vi "Pre-Loader.vi"(8 "error in (no error)":errorcluster) -> (0 "error out":errorcluster, 3 "Cancel?":bool)   [LabVIEW 2021, in "User Interface.lvlib"]
uses:
  User Interface.lvlib
  Pre-Loader Command.ctl
  CVT/Input Command.ctl
  Database/Database.lvlib
  DAQ Hardware/DAQ Hardware.lvlib
  DAQ IO/DAQ IO.lvlib
  ARINC/ARINC.lvlib
  S-Matrix/S-Matrix.lvlib
  DC PWS/DC PWS.lvlib
  DMM/DMM.lvlib
  Func Generator/Func Generator.lvlib
  Oscilloscope/Oscilloscope.lvlib
  Environment Chamber/Environment Chamber.lvlib
  CVT/CVT.lvlib
  CAN/CAN.lvlib
panel:
  out "Exit?":bool
  out "Title?":string="Pre-Loader"
  out "Msg":string
  out "Slider":i32(slide) scale=0.0..10.0
  in  "Stop":bool
  out "Time":string="Sat  8/3/2019  8:10:44 PM"
  # "21/511, Hosur Rd, Electronic City, Phase 1,Bengaluru, Karnataka 560100"
  # "21/511, Hosur Rd, Lavakusha Nagar, 1st Phase, Electronic City, Bengaluru, Karnataka 560100"
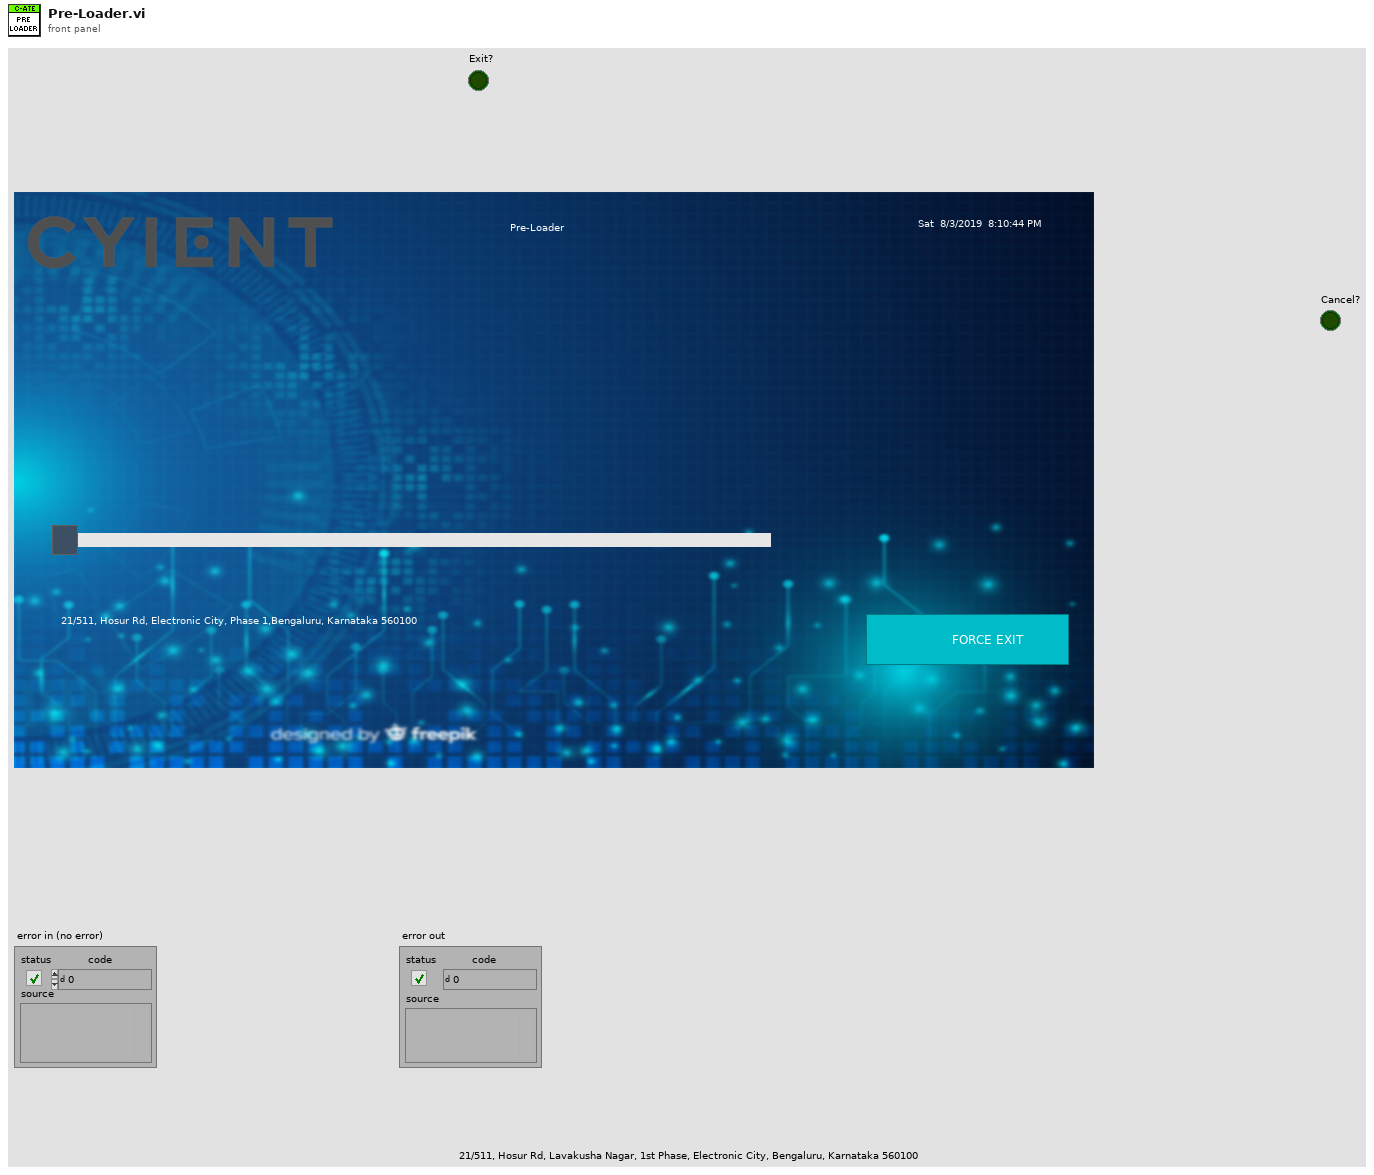
[diagram p1: front panel]
types:
  T1 = typedef "User Interface.lvlib/Pre-Loader Command.ctl" = enum16{"Init", "Check Database", "Check NI DAQ", "Check NI DIO", "Check CAN", "Check ARINC", "Check Matrix", "Check DC Power Supply", "Check DMM", "Check Function Gen", "Check Oscilloscope", "Check ESPEC", "Check CVT", "Exit"}
  T2 = typedef "CVT.lvlib/Input Command.ctl" = enum16{"DC PWS", "DMM", "FGEN", "Oscill", "NI DAQ", "NI DIO", "NI CAN", "ESPEC", "ARINC", "MATRIX", "CVT"}
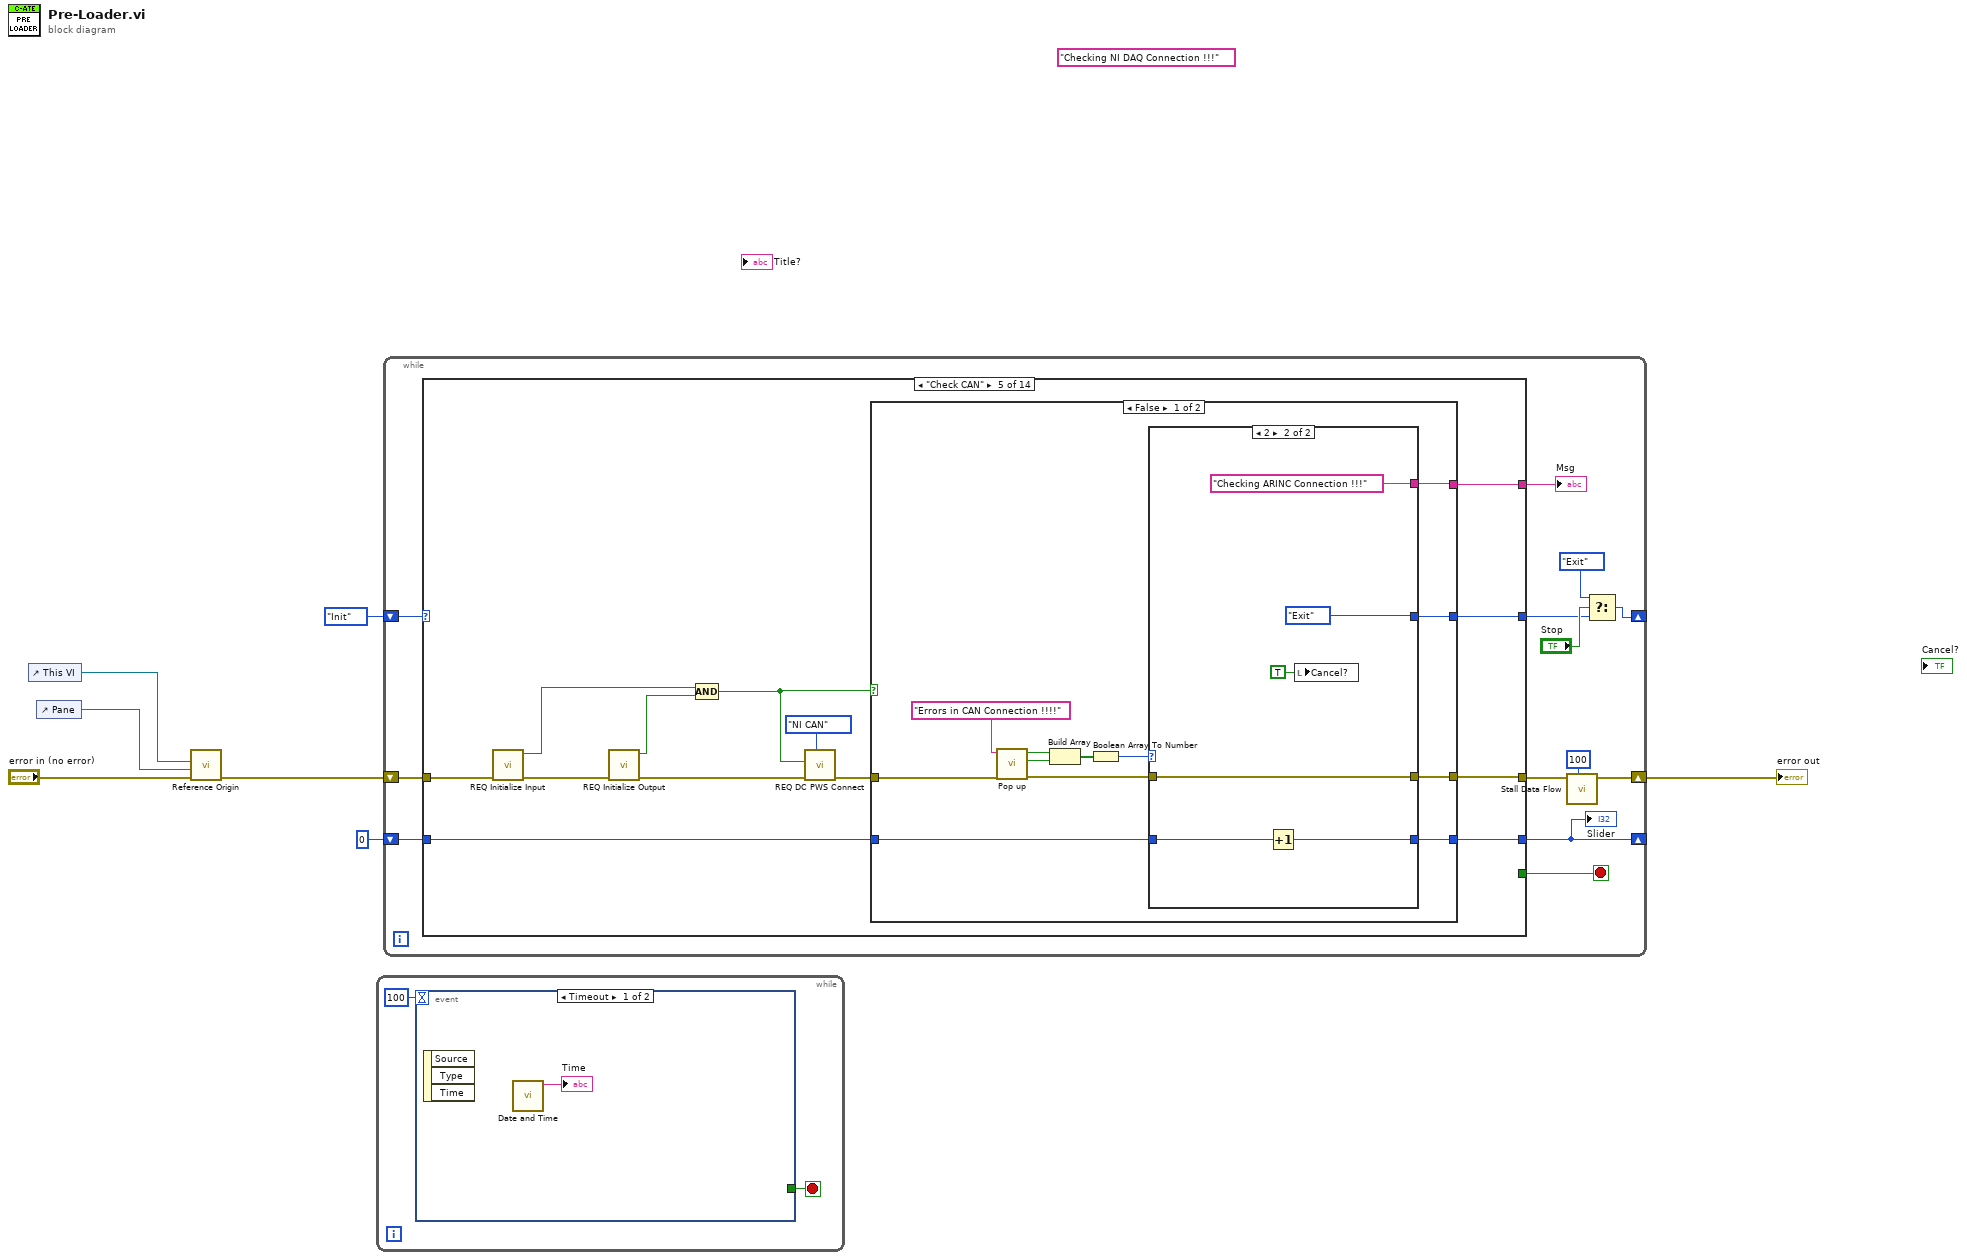
[diagram p0: block diagram]
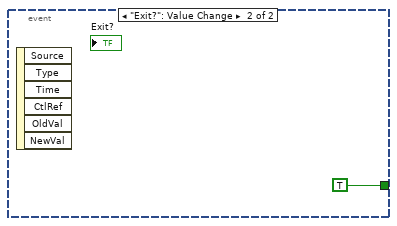
[diagram p2: hidden frame]
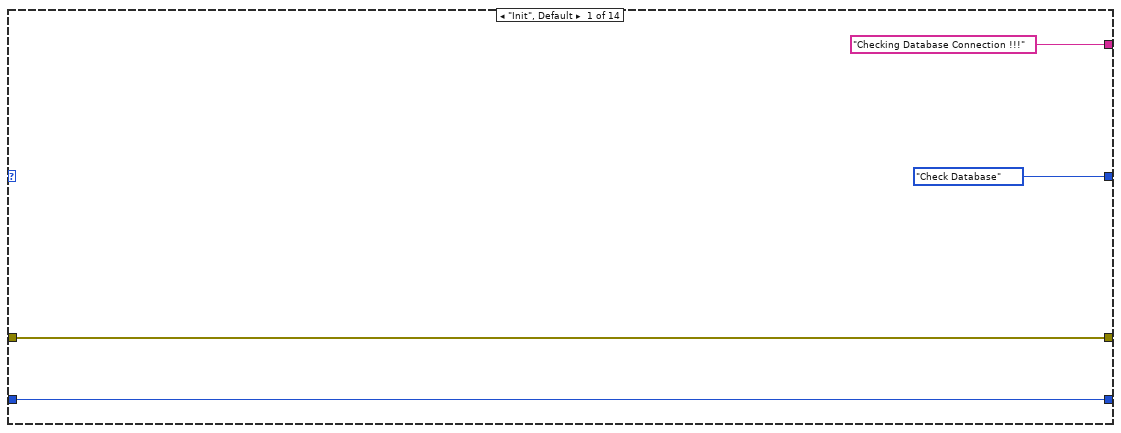
[diagram p3: hidden frame]
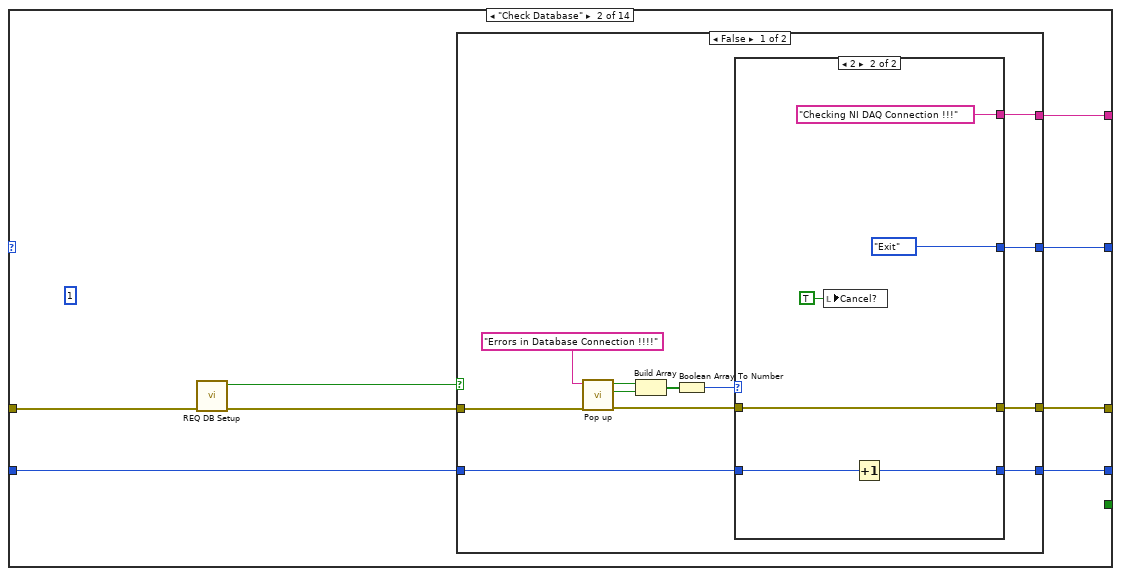
[diagram p4: hidden frame]
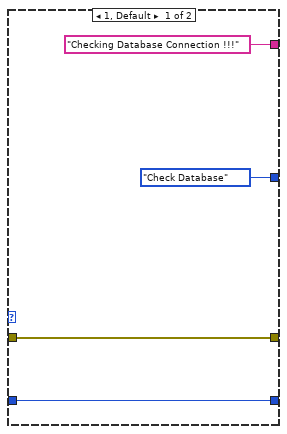
[diagram p5: hidden frame]
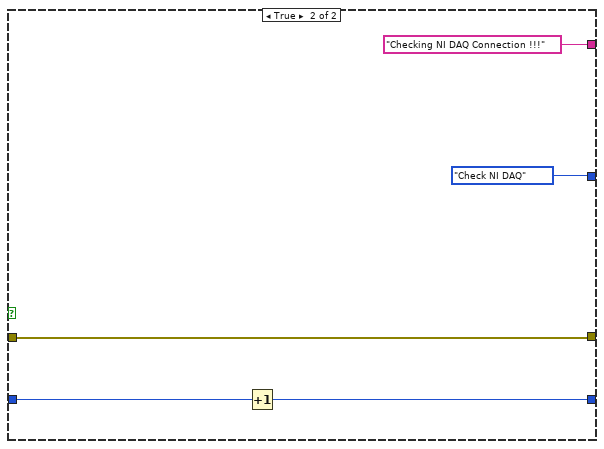
[diagram p6: hidden frame]
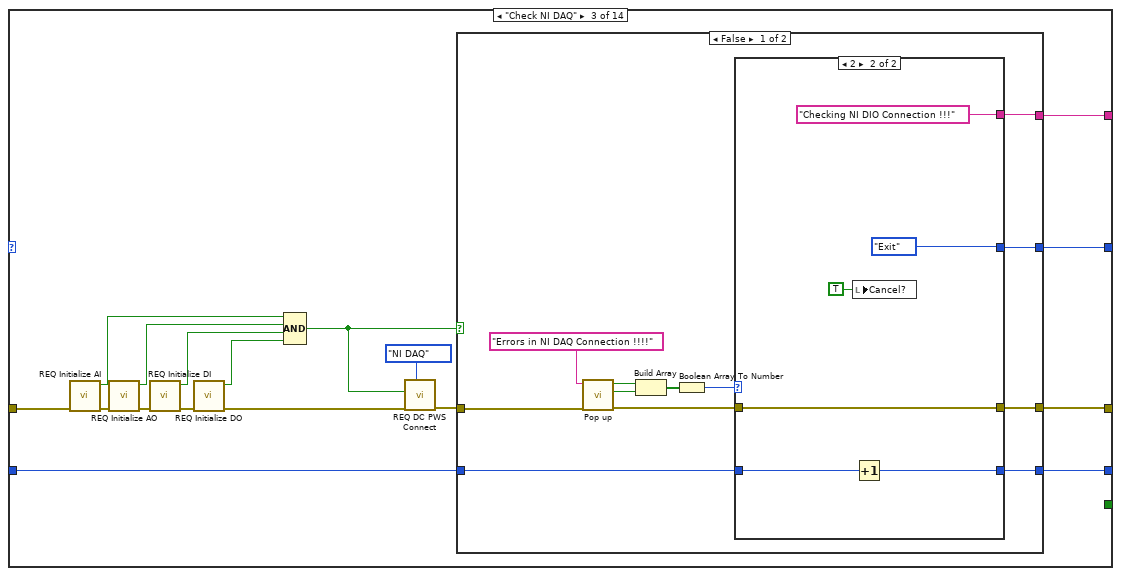
[diagram p7: hidden frame]
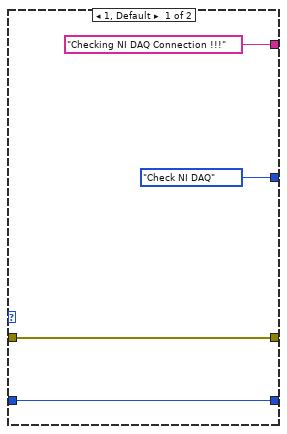
[diagram p8: hidden frame]
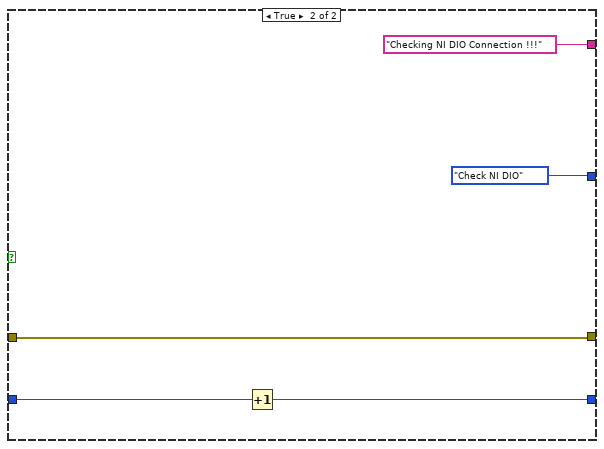
[diagram p9: hidden frame]
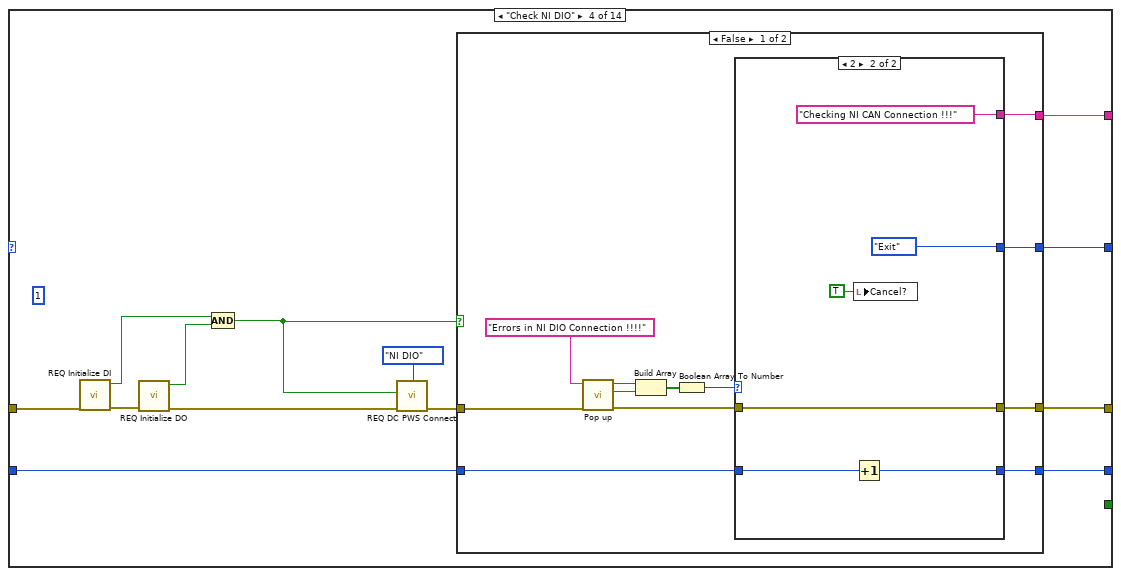
[diagram p10: hidden frame]
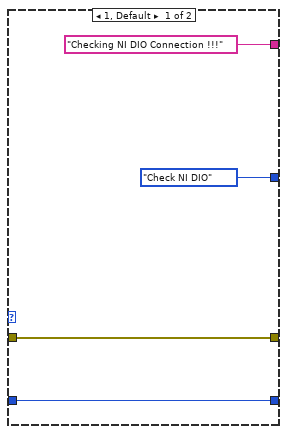
[diagram p11: hidden frame]
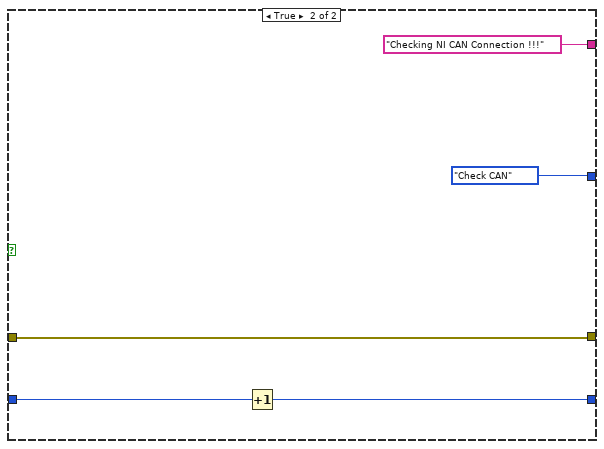
[diagram p12: hidden frame]
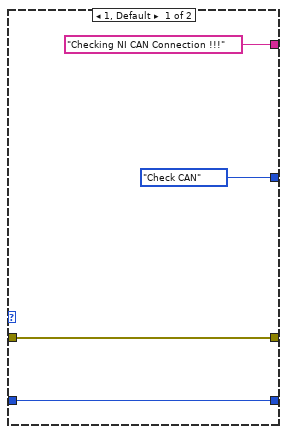
[diagram p13: hidden frame]
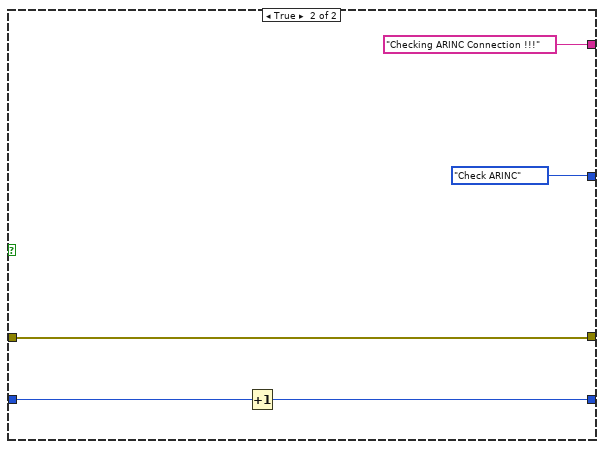
[diagram p14: hidden frame]
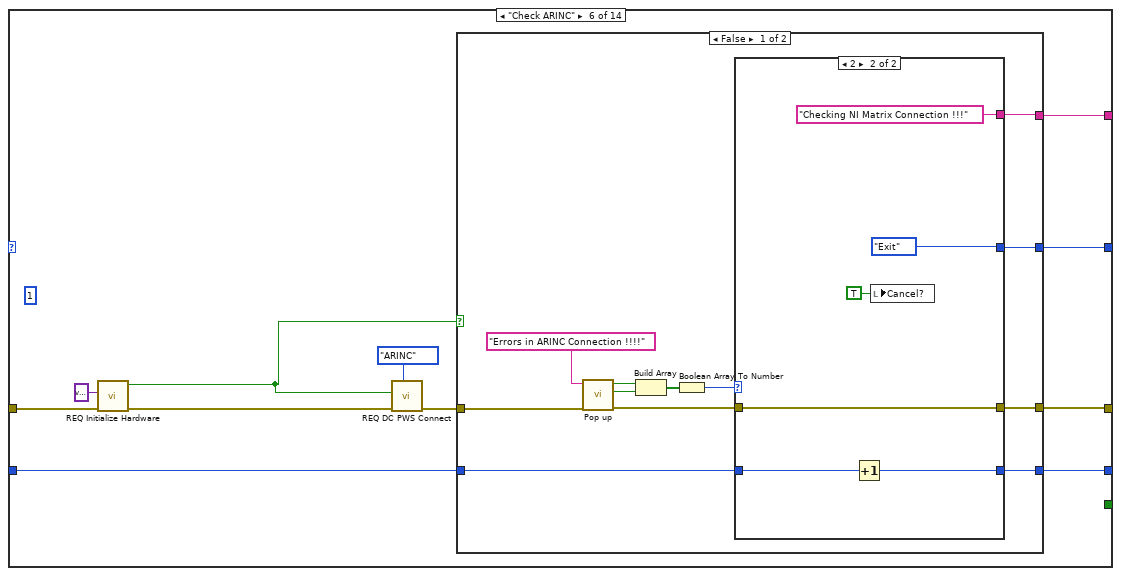
[diagram p15: hidden frame]
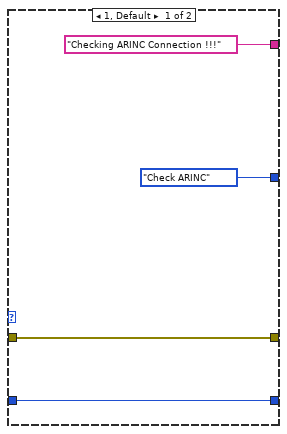
[diagram p16: hidden frame]
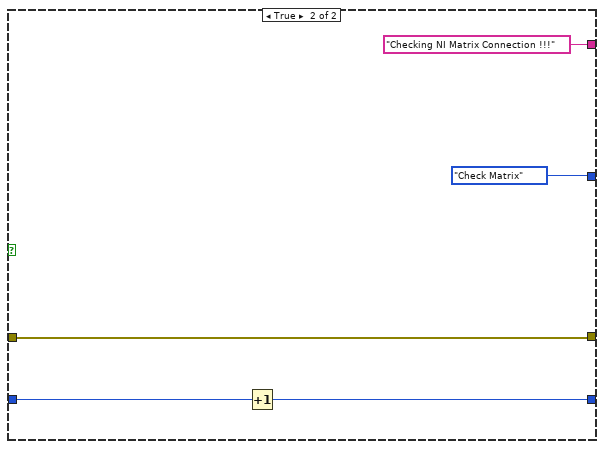
[diagram p17: hidden frame]
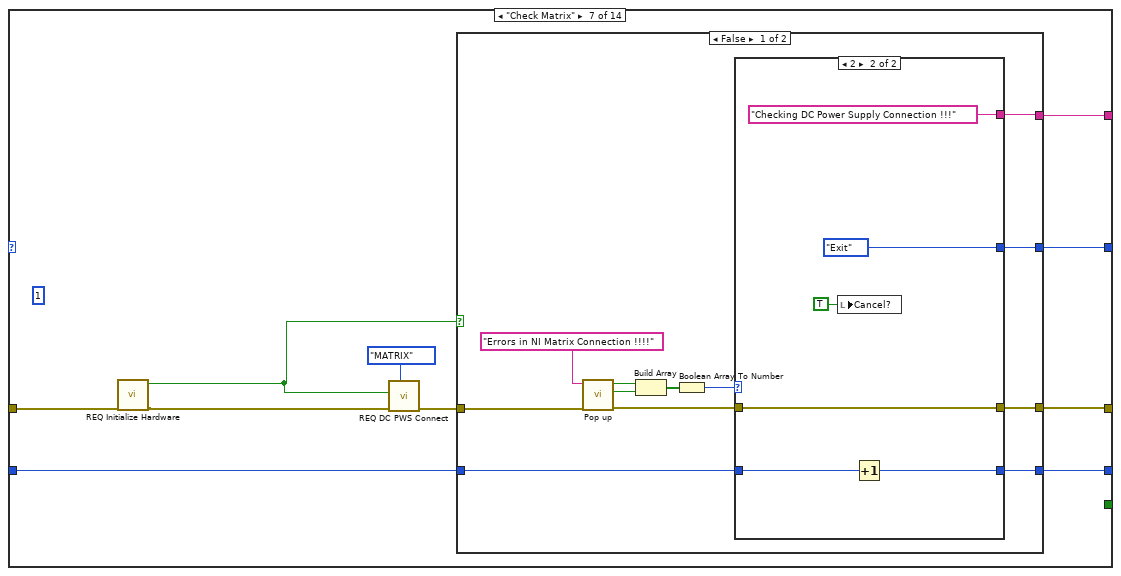
[diagram p18: hidden frame]
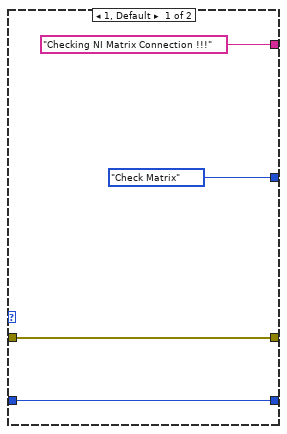
[diagram p19: hidden frame]
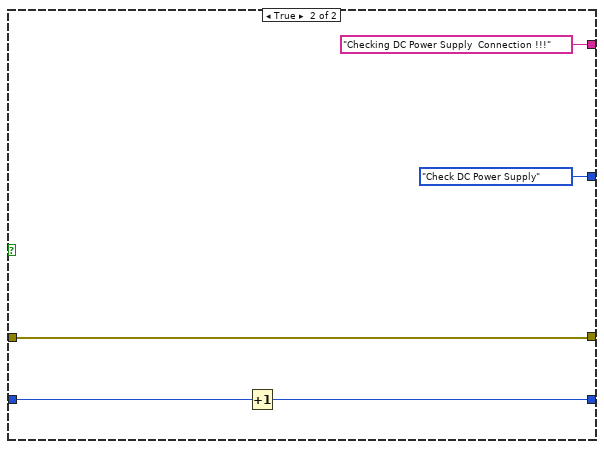
[diagram p20: hidden frame]
diagram:
  (unwired) "Checking NI DAQ Connection !!!"
  n1 = control-ref of="This VI"() -> (w6:refnum<vi>)
  n2 = control-ref of="Pane"() -> (w5:refnum<vi>)
  n3 = call "Reference Origin.vi"("error in (no error)"="error in (no error)", "Pane"=w5, "This VI"=w6) -> ("error out"=w4:errorcluster)  [unwired: 8 in]
  n4 = while {
    stop <- w8 stop-if-true
    n5 = event shown="[0] Timeout" {
      selector: _ -> [_ _]
      dyn-events: _ -> [_ _]
      timeout: 100 -> [_ _]
      tunnel: [_ TRUE] -> w8
      event Timeout {
        n6 = event-data() -> ()  [unwired: 1 in, 3 out]
        n7 = call "Date and Time.vi"() -> ("Current Time"=→"Time":string)  [unwired: 11 in]
      }
      event "Exit?": Value Change {
        n8 = event-data() -> ()  [unwired: 1 in, 6 out]
      }
    }
  }
  n9 = while {
    shift-right: [w20] -> _
    shift-left: Pre-Loader_Command."Init" -> [w24]
    shift-right: [w12] -> _
    shift-left: 0 -> [w13]
    shift-right: [w15] -> w3
    shift-left: w4 -> [w16]
    stop <- w18 stop-if-true
    n10 = case shown="\"Check CAN\"" w24 {
      tunnel: ["Checking Database Connection !!!" w29 w75 w115 w156 w193 w230 w267 w304 w341 w379 w417 w455 _] -> w23
      tunnel: [Pre-Loader_Command."Check Database" w30 w76 w116 w157 w194 w231 w268 w305 w342 w380 w418 w456 Pre-Loader_Command."Exit"] -> w21
      tunnel: [_ _ _ _ _ _ _ _ _ _ _ _ _ TRUE] -> w18
      tunnel: [w26 w33 w79 w119 w160 w197 w234 w271 w308 w345 w383 w421 w459 w487] -> w17
      tunnel: w16 -> [w26 w36 w80 w120 w153 w198 w235 w272 w309 w346 w384 w422 w452 w489]
      tunnel: w13 -> [w25 w32 w78 w118 w159 w196 w233 w270 w307 w344 w382 w420 w458 w491]
      tunnel: [w25 w31 w77 w117 w158 w195 w232 w269 w306 w343 w381 w419 w457 w491] -> w12
      frame "Init", Default {
      }
      frame "Check Database" {
        (unwired) 1
        n11 = call "REQ DB Setup.vi"("error in"=w36) -> ("error out"=w35:errorcluster, "Connect?"=w34:bool)  [unwired: 8 in, 1 out]
        n12 = case shown="False" w34 {
          tunnel: w35 -> [w48 w61]
          tunnel: [w39 w61] -> w33
          tunnel: w32 -> [w38 w63]
          tunnel: [w37 w62] -> w31
          tunnel: [w40 Pre-Loader_Command."Check NI DAQ"] -> w30
          tunnel: [w41 "Checking NI DAQ Connection !!!"] -> w29
          frame False {
            n13 = call "Pop up.vi"("error in (no error)"=w48, "Message In"="Errors in Database Connection !!!!") -> ("error out"=w42:errorcluster, "Next?"=w45:bool, "Retry?"=w46:bool)  [unwired: 7 in]
            n14 = Build Array(w46, w45) -> (w44:bool[])
            n15 = Boolean Array To Number(Boolean array=w44) -> (number=w43:u32)
            n16 = case shown="2" w43 {
              tunnel: w42 -> [w50 w56]
              tunnel: ["Checking Database Connection !!!" "Checking NI DAQ Connection !!!"] -> w41
              tunnel: [Pre-Loader_Command."Check Database" Pre-Loader_Command."Exit"] -> w40
              tunnel: [w50 w56] -> w39
              tunnel: w38 -> [w49 w55]
              tunnel: [w49 w54] -> w37
              frame 1, Default {
              }
              frame 2 {
                n17 = local write "Cancel?"(TRUE ("Cancel?")) -> ()
                n18 = Increment(x=w55) -> (x+1=w54:i32)
              }
            }
          }
          frame True {
            n19 = Increment(x=w63) -> (x+1=w62:i32)
          }
        }
      }
      frame "Check NI DAQ" {
        n20 = call "REQ Initialize AI.vi"("error in"=w80) -> ("error out"=w71:errorcluster, "Connect?"=w68:bool)  [unwired: 8 in, 1 out]
        n21 = call "REQ Initialize AO.vi"("error in"=w71) -> ("error out"=w70:errorcluster, "Connect?"=w67:bool)  [unwired: 8 in, 1 out]
        n22 = call "REQ Initialize DI.vi"("error in"=w70) -> ("error out"=w69:errorcluster, "Connect?"=w66:bool)  [unwired: 8 in, 1 out]
        n23 = call "REQ Initialize DO.vi"("error in"=w69) -> ("error out"=w73:errorcluster, "Connect?"=w65:bool)  [unwired: 8 in, 1 out]
        n24 = Compound Arithmetic op=AND(w68, w67, w66, w65) -> (w64:bool)
        n25 = call "REQ DC PWS Connect.vi"("Command"=Input_Command."NI DAQ", "error in"=w73, "Connect ?"=w64) -> ("error out"=w72:errorcluster)  [unwired: 8 in]
        n26 = case shown="False" w64 {
          tunnel: w72 -> [w92 w105]
          tunnel: [w83 w105] -> w79
          tunnel: w78 -> [w82 w107]
          tunnel: [w81 w106] -> w77
          tunnel: [w84 Pre-Loader_Command."Check NI DIO"] -> w76
          tunnel: [w85 "Checking NI DIO Connection !!!"] -> w75
          frame False {
            n27 = call "Pop up.vi"("error in (no error)"=w92, "Message In"="Errors in NI DAQ Connection !!!!") -> ("error out"=w86:errorcluster, "Next?"=w89:bool, "Retry?"=w90:bool)  [unwired: 7 in]
            n28 = Build Array(w90, w89) -> (w88:bool[])
            n29 = Boolean Array To Number(Boolean array=w88) -> (number=w87:u32)
            n30 = case shown="2" w87 {
              tunnel: w86 -> [w94 w100]
              tunnel: ["Checking NI DAQ Connection !!!" "Checking NI DIO Connection !!!"] -> w85
              tunnel: [Pre-Loader_Command."Check NI DAQ" Pre-Loader_Command."Exit"] -> w84
              tunnel: [w94 w100] -> w83
              tunnel: w82 -> [w93 w99]
              tunnel: [w93 w98] -> w81
              frame 1, Default {
              }
              frame 2 {
                n31 = local write "Cancel?"(TRUE ("Cancel?")) -> ()
                n32 = Increment(x=w99) -> (x+1=w98:i32)
              }
            }
          }
          frame True {
            n33 = Increment(x=w107) -> (x+1=w106:i32)
          }
        }
      }
      frame "Check NI DIO" {
        (unwired) 1
        n34 = call "REQ Initialize DI.vi"("error in"=w120) -> ("error out"=w110:errorcluster, "Connect?"=w108:bool)  [unwired: 8 in, 1 out]
        n35 = call "REQ Initialize DO.vi"("error in"=w110) -> ("error out"=w113:errorcluster, "Connect?"=w109:bool)  [unwired: 8 in, 1 out]
        n36 = Compound Arithmetic op=AND(w108, w109) -> (w111:bool)
        n37 = call "REQ DC PWS Connect.vi"("Command"=Input_Command."NI DIO", "error in"=w113, "Connect ?"=w111) -> ("error out"=w112:errorcluster)  [unwired: 8 in]
        n38 = case shown="False" w111 {
          tunnel: w112 -> [w132 w145]
          tunnel: [w123 w145] -> w119
          tunnel: w118 -> [w122 w147]
          tunnel: [w121 w146] -> w117
          tunnel: [w124 Pre-Loader_Command."Check CAN"] -> w116
          tunnel: [w125 "Checking NI CAN Connection !!!"] -> w115
          frame False {
            n39 = call "Pop up.vi"("error in (no error)"=w132, "Message In"="Errors in NI DIO Connection !!!!") -> ("error out"=w126:errorcluster, "Next?"=w129:bool, "Retry?"=w130:bool)  [unwired: 7 in]
            n40 = Build Array(w130, w129) -> (w128:bool[])
            n41 = Boolean Array To Number(Boolean array=w128) -> (number=w127:u32)
            n42 = case shown="2" w127 {
              tunnel: w126 -> [w134 w140]
              tunnel: ["Checking NI DIO Connection !!!" "Checking NI CAN Connection !!!"] -> w125
              tunnel: [Pre-Loader_Command."Check NI DIO" Pre-Loader_Command."Exit"] -> w124
              tunnel: [w134 w140] -> w123
              tunnel: w122 -> [w133 w139]
              tunnel: [w133 w138] -> w121
              frame 1, Default {
              }
              frame 2 {
                n43 = local write "Cancel?"(TRUE ("Cancel?")) -> ()
                n44 = Increment(x=w139) -> (x+1=w138:i32)
              }
            }
          }
          frame True {
            n45 = Increment(x=w147) -> (x+1=w146:i32)
          }
        }
      }
      frame "Check CAN" {
        n46 = call "REQ Initialize Input.vi"("error in"=w153) -> ("error out"=w152:errorcluster, "Connect?"=w150:bool)  [unwired: 8 in, 1 out]
        n47 = call "REQ Initialize Output.vi"("error in"=w152) -> ("error out"=w151:errorcluster, "Connect?"=w149:bool)  [unwired: 8 in, 1 out]
        n48 = Compound Arithmetic op=AND(w150, w149) -> (w148:bool)
        n49 = call "REQ DC PWS Connect.vi"("Command"=Input_Command."NI CAN", "error in"=w151, "Connect ?"=w148) -> ("error out"=w154:errorcluster)  [unwired: 8 in]
        n50 = case shown="False" w148 {
          tunnel: w154 -> [w172 w185]
          tunnel: [w163 w185] -> w160
          tunnel: w159 -> [w162 w187]
          tunnel: [w161 w186] -> w158
          tunnel: [w164 Pre-Loader_Command."Check ARINC"] -> w157
          tunnel: [w165 "Checking ARINC Connection !!!"] -> w156
          frame False {
            n51 = call "Pop up.vi"("error in (no error)"=w172, "Message In"="Errors in CAN Connection !!!!") -> ("error out"=w166:errorcluster, "Next?"=w169:bool, "Retry?"=w170:bool)  [unwired: 7 in]
            n52 = Build Array(w170, w169) -> (w168:bool[])
            n53 = Boolean Array To Number(Boolean array=w168) -> (number=w167:u32)
            n54 = case shown="2" w167 {
              tunnel: w166 -> [w174 w180]
              tunnel: ["Checking NI CAN Connection !!!" "Checking ARINC Connection !!!"] -> w165
              tunnel: [Pre-Loader_Command."Check CAN" Pre-Loader_Command."Exit"] -> w164
              tunnel: [w174 w180] -> w163
              tunnel: w162 -> [w173 w179]
              tunnel: [w173 w178] -> w161
              frame 1, Default {
              }
              frame 2 {
                n55 = Increment(x=w179) -> (x+1=w178:i32)
                n56 = local write "Cancel?"(TRUE ("Cancel?")) -> ()
              }
            }
          }
          frame True {
            n57 = Increment(x=w187) -> (x+1=w186:i32)
          }
        }
      }
      frame "Check ARINC" {
        (unwired) 1
        n58 = call "REQ Initialize Hardware.vi"("error in"=w198, "Connection Ref"=variant) -> ("error out"=w191:errorcluster, "Connect?"=w189:bool)  [unwired: 7 in, 1 out]
        n59 = call "REQ DC PWS Connect.vi"("Command"=Input_Command."ARINC", "error in"=w191, "Connect ?"=w189) -> ("error out"=w190:errorcluster)  [unwired: 8 in]
        n60 = case shown="False" w189 {
          tunnel: w190 -> [w210 w223]
          tunnel: [w201 w223] -> w197
          tunnel: w196 -> [w200 w225]
          tunnel: [w199 w224] -> w195
          tunnel: [w202 Pre-Loader_Command."Check Matrix"] -> w194
          tunnel: [w203 "Checking NI Matrix Connection !!!"] -> w193
          frame False {
            n61 = call "Pop up.vi"("error in (no error)"=w210, "Message In"="Errors in ARINC Connection !!!!") -> ("error out"=w204:errorcluster, "Next?"=w207:bool, "Retry?"=w208:bool)  [unwired: 7 in]
            n62 = Build Array(w208, w207) -> (w206:bool[])
            n63 = Boolean Array To Number(Boolean array=w206) -> (number=w205:u32)
            n64 = case shown="2" w205 {
              tunnel: w204 -> [w212 w218]
              tunnel: ["Checking ARINC Connection !!!" "Checking NI Matrix Connection !!!"] -> w203
              tunnel: [Pre-Loader_Command."Check ARINC" Pre-Loader_Command."Exit"] -> w202
              tunnel: [w212 w218] -> w201
              tunnel: w200 -> [w211 w217]
              tunnel: [w211 w216] -> w199
              frame 1, Default {
              }
              frame 2 {
                n65 = Increment(x=w217) -> (x+1=w216:i32)
                n66 = local write "Cancel?"(TRUE ("Cancel?")) -> ()
              }
            }
          }
          frame True {
            n67 = Increment(x=w225) -> (x+1=w224:i32)
          }
        }
      }
      frame "Check Matrix" {
        (unwired) 1
        n68 = call "REQ Initialize Hardware.vi"("error in"=w235) -> ("error out"=w228:errorcluster, "Connect?"=w226:bool)  [unwired: 8 in, 1 out]
        n69 = call "REQ DC PWS Connect.vi"("Command"=Input_Command."MATRIX", "error in"=w228, "Connect ?"=w226) -> ("error out"=w227:errorcluster)  [unwired: 8 in]
        n70 = case shown="False" w226 {
          tunnel: w227 -> [w247 w260]
          tunnel: [w238 w260] -> w234
          tunnel: w233 -> [w237 w262]
          tunnel: [w236 w261] -> w232
          tunnel: [w239 Pre-Loader_Command."Check DC Power Supply"] -> w231
          tunnel: [w240 "Checking DC Power Supply  Connection !!!"] -> w230
          frame False {
            n71 = call "Pop up.vi"("error in (no error)"=w247, "Message In"="Errors in NI Matrix Connection !!!!") -> ("error out"=w241:errorcluster, "Next?"=w244:bool, "Retry?"=w245:bool)  [unwired: 7 in]
            n72 = Build Array(w245, w244) -> (w243:bool[])
            n73 = Boolean Array To Number(Boolean array=w243) -> (number=w242:u32)
            n74 = case shown="2" w242 {
              tunnel: w241 -> [w249 w255]
              tunnel: ["Checking NI Matrix Connection !!!" "Checking DC Power Supply Connection !!!"] -> w240
              tunnel: [Pre-Loader_Command."Check Matrix" Pre-Loader_Command."Exit"] -> w239
              tunnel: [w249 w255] -> w238
              tunnel: w237 -> [w248 w254]
              tunnel: [w248 w253] -> w236
              frame 1, Default {
              }
              frame 2 {
                n75 = local write "Cancel?"(TRUE ("Cancel?")) -> ()
                n76 = Increment(x=w254) -> (x+1=w253:i32)
              }
            }
          }
          frame True {
            n77 = Increment(x=w262) -> (x+1=w261:i32)
          }
        }
      }
      frame "Check DC Power Supply" {
        (unwired) 1
        n78 = call "REQ Initialize Hardware.vi"("error in"=w272) -> ("error out"=w265:errorcluster, "Connect?"=w263:bool)  [unwired: 8 in, 1 out]
        n79 = call "REQ DC PWS Connect.vi"("Command"=Input_Command."DC PWS", "error in"=w265, "Connect ?"=w263) -> ("error out"=w264:errorcluster)  [unwired: 8 in]
        n80 = case shown="False" w263 {
          tunnel: w264 -> [w284 w297]
          tunnel: [w275 w297] -> w271
          tunnel: w270 -> [w274 w299]
          tunnel: [w273 w298] -> w269
          tunnel: [w276 Pre-Loader_Command."Check DMM"] -> w268
          tunnel: [w277 "Checking DMM  Connection !!!"] -> w267
          frame False {
            n81 = call "Pop up.vi"("error in (no error)"=w284, "Message In"="Errors in DC Power Supply Connection !!!!") -> ("error out"=w278:errorcluster, "Next?"=w281:bool, "Retry?"=w282:bool)  [unwired: 7 in]
            n82 = Build Array(w282, w281) -> (w280:bool[])
            n83 = Boolean Array To Number(Boolean array=w280) -> (number=w279:u32)
            n84 = case shown="2" w279 {
              tunnel: w278 -> [w286 w292]
              tunnel: ["Checking DC Power Supply Connection !!!" "Checking DMM Connection !!!"] -> w277
              tunnel: [Pre-Loader_Command."Check DC Power Supply" Pre-Loader_Command."Exit"] -> w276
              tunnel: [w286 w292] -> w275
              tunnel: w274 -> [w285 w291]
              tunnel: [w285 w290] -> w273
              frame 1, Default {
              }
              frame 2 {
                n85 = local write "Cancel?"(TRUE ("Cancel?")) -> ()
                n86 = Increment(x=w291) -> (x+1=w290:i32)
              }
            }
          }
          frame True {
            n87 = Increment(x=w299) -> (x+1=w298:i32)
          }
        }
      }
      frame "Check DMM" {
        (unwired) 1
        n88 = call "REQ Initialize Hardware.vi"("error in"=w309) -> ("error out"=w302:errorcluster, "Connect?"=w300:bool)  [unwired: 8 in, 1 out]
        n89 = call "REQ DC PWS Connect.vi"("Command"=Input_Command."DMM", "error in"=w302, "Connect ?"=w300) -> ("error out"=w301:errorcluster)  [unwired: 8 in]
        n90 = case shown="False" w300 {
          tunnel: w301 -> [w321 w334]
          tunnel: [w312 w334] -> w308
          tunnel: w307 -> [w311 w336]
          tunnel: [w310 w335] -> w306
          tunnel: [w313 Pre-Loader_Command."Check Function Gen"] -> w305
          tunnel: [w314 "Checking Function Generator  Connection !!!"] -> w304
          frame False {
            n91 = call "Pop up.vi"("error in (no error)"=w321, "Message In"="Errors in DMM Connection !!!!") -> ("error out"=w315:errorcluster, "Next?"=w318:bool, "Retry?"=w319:bool)  [unwired: 7 in]
            n92 = Build Array(w319, w318) -> (w317:bool[])
            n93 = Boolean Array To Number(Boolean array=w317) -> (number=w316:u32)
            n94 = case shown="2" w316 {
              tunnel: w315 -> [w323 w329]
              tunnel: ["Checking DMM Connection !!!" "Checking Function Generator Connection !!!"] -> w314
              tunnel: [Pre-Loader_Command."Check DMM" Pre-Loader_Command."Exit"] -> w313
              tunnel: [w323 w329] -> w312
              tunnel: w311 -> [w322 w328]
              tunnel: [w322 w327] -> w310
              frame 1, Default {
              }
              frame 2 {
                n95 = Increment(x=w328) -> (x+1=w327:i32)
                n96 = local write "Cancel?"(TRUE ("Cancel?")) -> ()
              }
            }
          }
          frame True {
            n97 = Increment(x=w336) -> (x+1=w335:i32)
          }
        }
      }
      frame "Check Function Gen" {
        (unwired) 1
        n98 = call "REQ Initialize Hardware.vi"("error in"=w346) -> ("error out"=w339:errorcluster, "Connect?"=w337:bool)  [unwired: 8 in, 1 out]
        n99 = call "REQ DC PWS Connect.vi"("Command"=Input_Command."FGEN", "error in"=w339, "Connect ?"=w337) -> ("error out"=w338:errorcluster)  [unwired: 8 in]
        n100 = case shown="False" w337 {
          tunnel: w338 -> [w358 w371]
          tunnel: [w349 w371] -> w345
          tunnel: w344 -> [w348 w373]
          tunnel: [w347 w372] -> w343
          tunnel: [w350 Pre-Loader_Command."Check Oscilloscope"] -> w342
          tunnel: [w351 "Checking Oscilloscope  Connection !!!"] -> w341
          frame False {
            n101 = call "Pop up.vi"("error in (no error)"=w358, "Message In"="Errors in Function Generator Connection !!!!") -> ("error out"=w352:errorcluster, "Next?"=w355:bool, "Retry?"=w356:bool)  [unwired: 7 in]
            n102 = Build Array(w356, w355) -> (w354:bool[])
            n103 = Boolean Array To Number(Boolean array=w354) -> (number=w353:u32)
            n104 = case shown="2" w353 {
              tunnel: w352 -> [w360 w366]
              tunnel: ["Checking Function Generator Connection !!!" "Checking Oscilloscope Connection !!!"] -> w351
              tunnel: [Pre-Loader_Command."Check Function Gen" Pre-Loader_Command."Exit"] -> w350
              tunnel: [w360 w366] -> w349
              tunnel: w348 -> [w359 w365]
              tunnel: [w359 w364] -> w347
              frame 1, Default {
              }
              frame 2 {
                n105 = local write "Cancel?"(TRUE ("Cancel?")) -> ()
                n106 = Increment(x=w365) -> (x+1=w364:i32)
              }
            }
          }
          frame True {
            n107 = Increment(x=w373) -> (x+1=w372:i32)
          }
        }
      }
      frame "Check Oscilloscope" {
        (unwired) 1
        n108 = call "REQ Initialize Hardware.vi"("error in"=w384, "Connection Ref"=variant) -> ("error out"=w377:errorcluster, "Connect?"=w375:bool)  [unwired: 7 in, 1 out]
        n109 = call "REQ DC PWS Connect.vi"("Command"=Input_Command."Oscill", "error in"=w377, "Connect ?"=w375) -> ("error out"=w376:errorcluster)  [unwired: 8 in]
        n110 = case shown="False" w375 {
          tunnel: w376 -> [w396 w409]
          tunnel: [w387 w409] -> w383
          tunnel: w382 -> [w386 w411]
          tunnel: [w385 w410] -> w381
          tunnel: [w388 Pre-Loader_Command."Check ESPEC"] -> w380
          tunnel: [w389 "Checking Environment Chamber  Connection !!!"] -> w379
          frame False {
            n111 = call "Pop up.vi"("error in (no error)"=w396, "Message In"="Errors in Oscilloscope Connection !!!!") -> ("error out"=w390:errorcluster, "Next?"=w393:bool, "Retry?"=w394:bool)  [unwired: 7 in]
            n112 = Build Array(w394, w393) -> (w392:bool[])
            n113 = Boolean Array To Number(Boolean array=w392) -> (number=w391:u32)
            n114 = case shown="2" w391 {
              tunnel: w390 -> [w398 w404]
              tunnel: ["Checking Oscilloscope Connection !!!" "Checking Environment Chamber Connection !!!"] -> w389
              tunnel: [Pre-Loader_Command."Check Oscilloscope" Pre-Loader_Command."Exit"] -> w388
              tunnel: [w398 w404] -> w387
              tunnel: w386 -> [w397 w403]
              tunnel: [w397 w402] -> w385
              frame 1, Default {
              }
              frame 2 {
                n115 = Increment(x=w403) -> (x+1=w402:i32)
                n116 = local write "Cancel?"(TRUE ("Cancel?")) -> ()
              }
            }
          }
          frame True {
            n117 = Increment(x=w411) -> (x+1=w410:i32)
          }
        }
      }
      frame "Check ESPEC" {
        (unwired) 1
        n118 = call "REQ Initialize Hardware.vi"("error in"=w422, "Connection Ref"=variant) -> ("error out"=w415:errorcluster, "Connect?"=w413:bool)  [unwired: 7 in, 1 out]
        n119 = call "REQ DC PWS Connect.vi"("Command"=Input_Command."ESPEC", "error in"=w415, "Connect ?"=w413) -> ("error out"=w414:errorcluster)  [unwired: 8 in]
        n120 = case shown="False" w413 {
          tunnel: w414 -> [w434 w447]
          tunnel: [w425 w447] -> w421
          tunnel: w420 -> [w424 w449]
          tunnel: [w423 w448] -> w419
          tunnel: [w426 Pre-Loader_Command."Check CVT"] -> w418
          tunnel: [w427 "Checking CVT  Connection !!!"] -> w417
          frame False {
            n121 = call "Pop up.vi"("error in (no error)"=w434, "Message In"="Errors in Environment Chamber Connection !!!!") -> ("error out"=w428:errorcluster, "Next?"=w431:bool, "Retry?"=w432:bool)  [unwired: 7 in]
            n122 = Build Array(w432, w431) -> (w430:bool[])
            n123 = Boolean Array To Number(Boolean array=w430) -> (number=w429:u32)
            n124 = case shown="2" w429 {
              tunnel: w428 -> [w436 w443]
              tunnel: ["Checking Environment Chamber Connection !!!" "Closing Pre-Loader !!!"] -> w427
              tunnel: [Pre-Loader_Command."Check ESPEC" Pre-Loader_Command."Exit"] -> w426
              tunnel: [w436 w443] -> w425
              tunnel: w424 -> [w435 w442]
              tunnel: [w435 w441] -> w423
              frame 1, Default {
              }
              frame 2 {
                n125 = Increment(x=w442) -> (x+1=w441:i32)
                n126 = local write "Cancel?"(TRUE ("Cancel?")) -> ()
              }
            }
          }
          frame True {
            n127 = Increment(x=w449) -> (x+1=w448:i32)
          }
        }
      }
      frame "Check CVT" {
        (unwired) 1
        n128 = call "REQ Initializ CVT.vi"("error in"=w452) -> ("error out"=w451:errorcluster, "Connect?"=w450:bool)  [unwired: 8 in, 1 out]
        n129 = call "REQ DC PWS Connect.vi"("Command"=Input_Command."CVT", "error in"=w451, "Connect ?"=w450) -> ("error out"=w453:errorcluster)  [unwired: 8 in]
        n130 = case shown="False" w450 {
          tunnel: w453 -> [w471 w484]
          tunnel: [w462 w484] -> w459
          tunnel: w458 -> [w461 w486]
          tunnel: [w460 w485] -> w457
          tunnel: [w463 Pre-Loader_Command."Exit"] -> w456
          tunnel: [w464 "Closing Pre-Loader !!!"] -> w455
          frame False {
            n131 = call "Pop up.vi"("error in (no error)"=w471, "Message In"="Errors in CVT Connection !!!!") -> ("error out"=w465:errorcluster, "Next?"=w468:bool, "Retry?"=w469:bool)  [unwired: 7 in]
            n132 = Build Array(w469, w468) -> (w467:bool[])
            n133 = Boolean Array To Number(Boolean array=w467) -> (number=w466:u32)
            n134 = case shown="2" w466 {
              tunnel: w465 -> [w473 w480]
              tunnel: ["Checking Environment Chamber Connection !!!" "Closing Pre-Loader !!!"] -> w464
              tunnel: [Pre-Loader_Command."Check ESPEC" Pre-Loader_Command."Exit"] -> w463
              tunnel: [w473 w480] -> w462
              tunnel: w461 -> [w472 w479]
              tunnel: [w472 w478] -> w460
              frame 1, Default {
              }
              frame 2 {
                n135 = Increment(x=w479) -> (x+1=w478:i32)
                n136 = local write "Cancel?"(TRUE ("Cancel?")) -> ()
              }
            }
          }
          frame True {
            n137 = Increment(x=w486) -> (x+1=w485:i32)
          }
        }
      }
      frame "Exit" {
        n138 = property on="Exit?" class="Bool (strict)"(error in=w489, "Val(Sgnl)"=TRUE ("Value (Signaling)")) -> (error out=w487:errorcluster)  [unwired: 1 in, 1 out]
      }
    }
    "Msg" <- w23
    "Slider" <- w12
    n139 = call "Stall Data Flow.vi"("milliseconds to wait"=u32 100, "error in (no error)"=w17) -> ("error out"=w15:errorcluster)  [unwired: 9 in]
    n140 = Select(t=Pre-Loader_Command."Exit", s="Stop", f=w21) -> (s? t:f=w20:T1)
  }
  "error out" <- w3
